vi "PrimaryInterfaceGetState.vi"(8 "PrimaryInterface":refnum<k24>, 11 "error in":errorcluster) -> (0 "Connected":bool, 3 "error out":errorcluster)   [LabVIEW 2021, in "UnderAutomation.UniversalRobots.lvlib"]
uses:
  UnderAutomation.UniversalRobots.lvlib
  C:/Users/fg/Documents/UniversalRobots.vi/LabVIEW_2024/UnderAutomation.UniversalRobots/lib/UnderAutomation.UniversalRobots.dll
  LabVIEW_2024/UnderAutomation.UniversalRobots/lib/UnderAutomation.UniversalRobots.dll
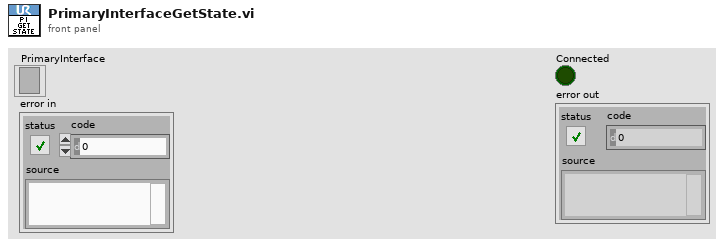
[diagram p1: front panel]
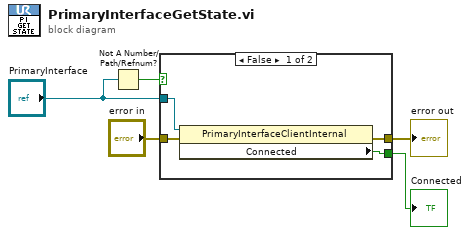
[diagram p0: block diagram]
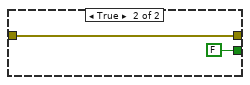
[diagram p2: hidden frame]
diagram:
  n1 = Not A Number/Path/Refnum?(number/path/refnum="PrimaryInterface") -> (NaN/Path/Refnum?=w1:bool)
  n2 = case shown="False" w1 {
    tunnel: [w9 FALSE ("Connected")] -> w5
    tunnel: "error in" -> [w8 w11]
    tunnel: [w7 w11] -> w3
    tunnel: "PrimaryInterface" -> [w6 _]
    frame False {
      n3 = property class="PrimaryInterfaceClientInternal"(reference=w6, error in=w8) -> (error out=w7:errorcluster, "Connected"=w9:bool)  [unwired: 1 out]
    }
    frame True {
    }
  }
  "Connected" <- w5
  "error out" <- w3
